vi "Write Aalborg GFC17 Connections.vi"(8 "error in (no error)":errorcluster, 10 "Aalborg GFC17 Connections":T1={"flow rate setpoint channel"="cDAQ1Mod3/ao0", "flow rate reading channel"="cDAQ1Mod1/ai4", "valve channel"="cDAQ1Mod3/ao1"}, 11 "Aalborg GFC17 in":refnum<class "Aalborg GFC17.lvclass">) -> (0 "error out":errorcluster, 3 "Aalborg GFC17 out":refnum<class "Aalborg GFC17.lvclass">)   [LabVIEW 2011, in "Aalborg GFC17.lvclass"]
uses:
  Aalborg GFC17.lvclass
  Aalborg GFC17 Connections.ctl
  Aalborg GFC17.lvclass/Aalborg GFC17.ctl
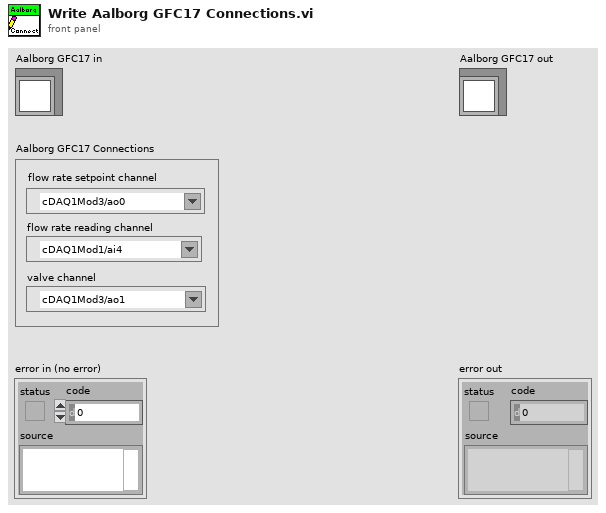
[diagram p1: front panel]
types:
  T1 = typedef "Aalborg GFC17.lvclass/Aalborg GFC17 Connections.ctl" = cluster{"flow rate setpoint channel":tag, "flow rate reading channel":tag, "valve channel":tag}
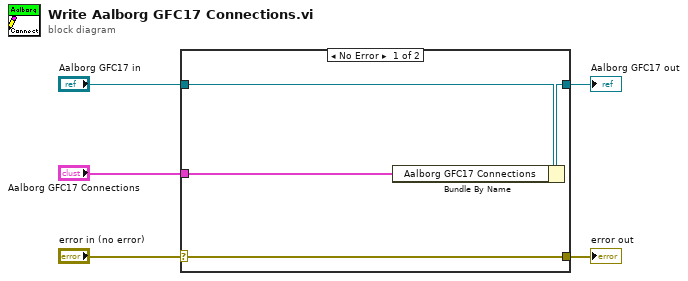
[diagram p0: block diagram]
diagram:
  n1 = case shown="No Error" "error in (no error)" {
    selector: "error in (no error)" -> [w9 w10]
    tunnel: [w9 w10] -> w4
    tunnel: [w7 w11] -> w2
    tunnel: "Aalborg GFC17 in" -> [w8 w11]
    tunnel: "Aalborg GFC17 Connections" -> [w6 _]
    frame No Error {
      n2 = Bundle By Name(cluster=w8, "Aalborg GFC17 Connections"=w6) -> (w7:refnum<class "Aalborg GFC17.lvclass">)
    }
    frame Error {
    }
  }
  "error out" <- w4
  "Aalborg GFC17 out" <- w2
